vi "Drive Train Charts.vi"() -> ()   [LabVIEW 2016]
uses:
  <vilib>/Rock Robotics/Network Tables/NT Read Number.vi
panel:
  out "Right Target":dbl(graph)
  out "Right Throttle":dbl(graph)
  out "Right Velocity":dbl(graph)
  out "Right Current":dbl(graph)
  out "Left Target":dbl(graph)
  out "Left Throttle":dbl(graph)
  out "Left Velocity":dbl(graph)
  out "Left Current":dbl(graph)
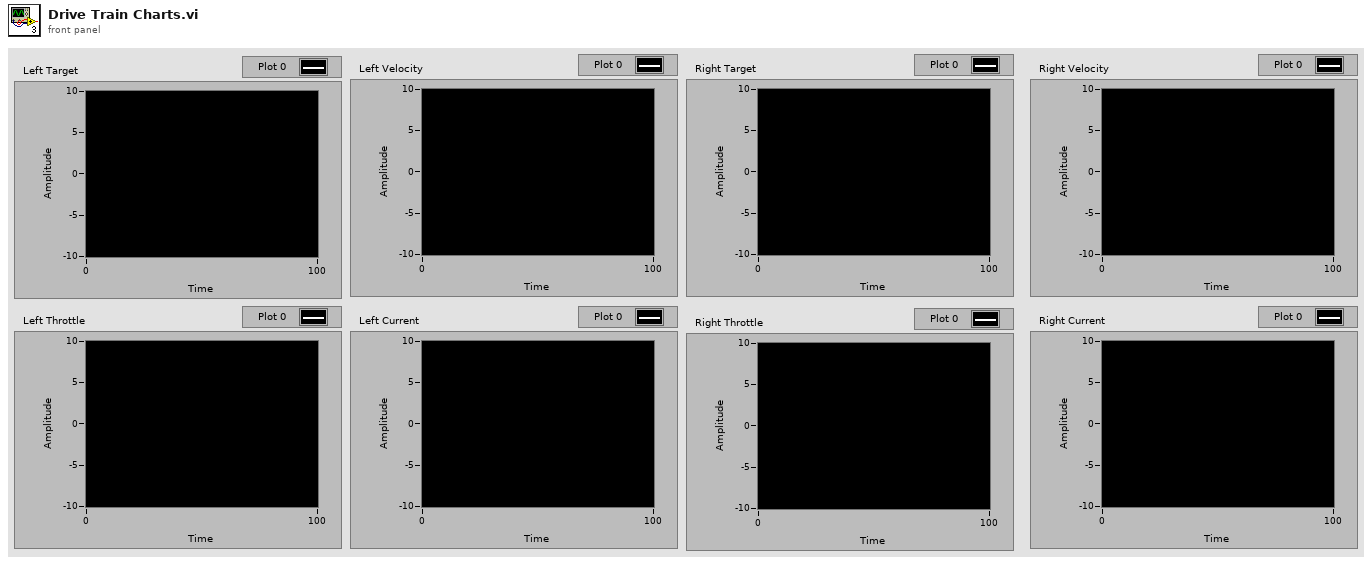
[diagram p1: front panel]
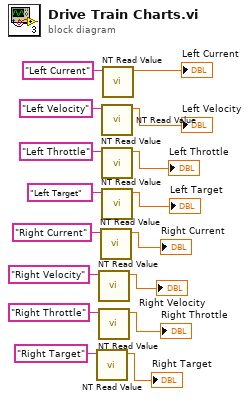
[diagram p0: block diagram]
diagram:
  n1 = call-poly <vilib>:"NT Read Value.vi"("Name"="Right Target") -> ("Numeric"=→"Right Target":dbl)  [unwired: 9 in, 1 out]
  n2 = call-poly <vilib>:"NT Read Value.vi"("Name"="Right Velocity") -> ("Numeric"=→"Right Velocity":dbl)  [unwired: 9 in, 1 out]
  n3 = call-poly <vilib>:"NT Read Value.vi"("Name"="Right Throttle") -> ("Numeric"=→"Right Throttle":dbl)  [unwired: 9 in, 1 out]
  n4 = call-poly <vilib>:"NT Read Value.vi"("Name"="Right Current") -> ("Numeric"=→"Right Current":dbl)  [unwired: 9 in, 1 out]
  n5 = call-poly <vilib>:"NT Read Value.vi"("Name"="Left Velocity") -> ("Numeric"=→"Left Velocity":dbl)  [unwired: 9 in, 1 out]
  n6 = call-poly <vilib>:"NT Read Value.vi"("Name"="Left Throttle") -> ("Numeric"=→"Left Throttle":dbl)  [unwired: 9 in, 1 out]
  n7 = call-poly <vilib>:"NT Read Value.vi"("Name"="Left Target") -> ("Numeric"=→"Left Target":dbl)  [unwired: 9 in, 1 out]
  n8 = call-poly <vilib>:"NT Read Value.vi"("Name"="Left Current") -> ("Numeric"=→"Left Current":dbl)  [unwired: 9 in, 1 out]
